vi "New Interface.vi"(5 "FIFO Options":T1, 6 "id (0)":i32, 7 "fifo/queue depths (10)":u32=10, 8 "error in (no error)":errorcluster, 10 "error size (512 B)":T2=enum."512-byte", 11 "Interface type":refnum<class "Interface.lvclass">) -> (0 "error out":errorcluster, 3 "Interface":refnum<class "Interface.lvclass">)   [LabVIEW 2017, in "DSF Core.lvlib" / "Interface.lvclass"]
uses:
  Interface.lvclass
  Error Queue Sizes.ctl
  Typedefs/DSF FIFO Options.ctl
  Interface.lvclass/Interface.ctl
  DSF Core.lvlib
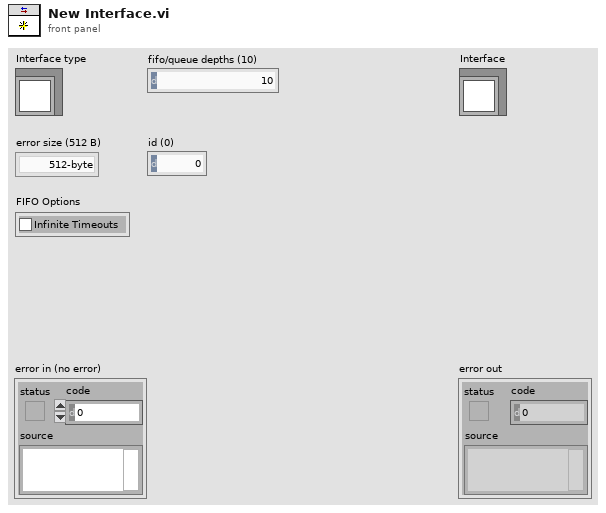
[diagram p1: front panel]
types:
  T1 = typedef "DSF Core.lvlib/DSF FIFO Options.ctl" = cluster{"Infinite Timeouts":bool}
  T2 = typedef "DSF Core.lvlib/Interface.lvclass/Error Queue Sizes.ctl" = enum16{"256-byte", "512-byte", "1024-byte"}
  T3 = typedef "DSF Core.lvlib/Interface.lvclass/RT FIFO Ref.ctl" = refnum<k33>
  T4 = typedef "DSF Core.lvlib/Interface.lvclass/Error Queue Ref.ctl" = refnum<queue>
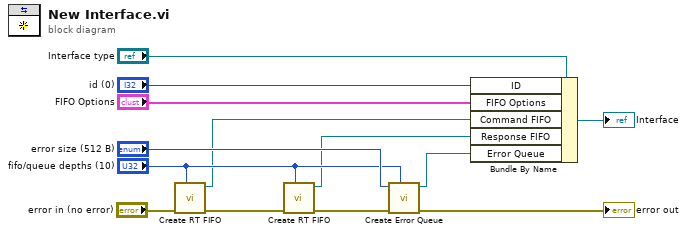
[diagram p0: block diagram]
diagram:
  n1 = call "Create RT FIFO.vi"("size (10)"="fifo/queue depths (10)", "error in (no error)"="error in (no error)") -> ("error out"=w11:errorcluster, "RT FIFO"=w3:T3)  [unwired: 8 in]
  n2 = call "Create RT FIFO.vi"("size (10)"="fifo/queue depths (10)", "error in (no error)"=w11) -> ("error out"=w10:errorcluster, "RT FIFO"=w2:T3)  [unwired: 8 in]
  n3 = call "Create Error Queue.vi"("max queue size (10)"="fifo/queue depths (10)", "error in (no error)"=w10, "error size"="error size (512 B)") -> ("error out"=→"error out":errorcluster, "Error Queue"=w1:T4)  [unwired: 7 in]
  n4 = Bundle By Name(cluster="Interface type", "ID"="id (0)", "FIFO Options"="FIFO Options", "Command FIFO"=w3, "Response FIFO"=w2, "Error Queue"=w1) -> (→"Interface":refnum<class "Interface.lvclass">)
